vi "runScript.vi"(6 "timeStamp":string, 8 "error in (no error)":errorcluster, 9 "Path":path, 10 "CompiledScript":T1, 11 "AtomChipHWC in":refnum<class "AtomChipHWC.lvclass">) -> (0 "error out":errorcluster, 3 "AtomChipHWC out":refnum<class "AtomChipHWC.lvclass">)   [LabVIEW 2011, in "Hardware.lvlib" / "HWControllers.lvlib" / "AtomChipHWC.lvclass"]
uses:
  AtomChipHWC.lvclass
  Tools/SettingsProcessors/ScriptListCompiler/ScriptListCompiler.lvclass
  Channels/VoltOutput/AnalogOutput.lvclass
  Channels/Digital/DigitalOutput.lvclass
  Channels/DDSOutput/Generic/DDSOutput.lvclass
  AtomChipHWC.lvclass/AtomChipHWC.ctl
  HWController.lvclass
  HardwareConfiguration/HWConfiguration.lvclass
panel:
  out "Analog time":dbl
  out "DDS time":dbl
  out "Digital Time":dbl
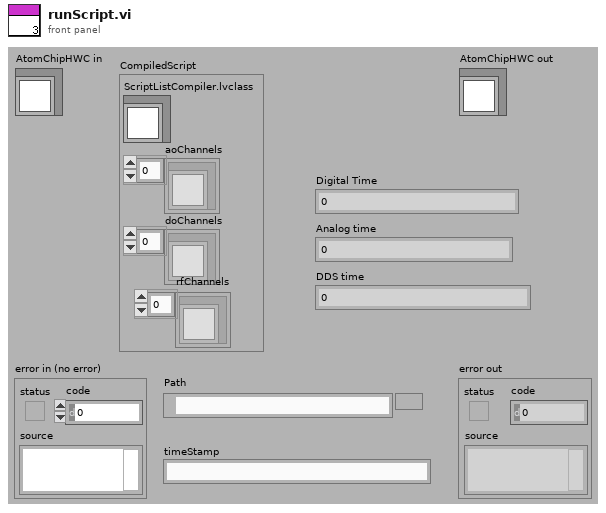
[diagram p1: front panel]
types:
  T1 = cluster{"ScriptListCompiler.lvclass":refnum<class "ScriptListCompiler.lvclass">, "aoChannels":refnum<class "AnalogOutput.lvclass">[], "doChannels":refnum<class "DigitalOutput.lvclass">[], "rfChannels":refnum<class "DDSOutput.lvclass">[]}
  T2 = enum16{"Ready", "Compiling", "Configured", "Running", "Stopping", "Unresolved Error"}
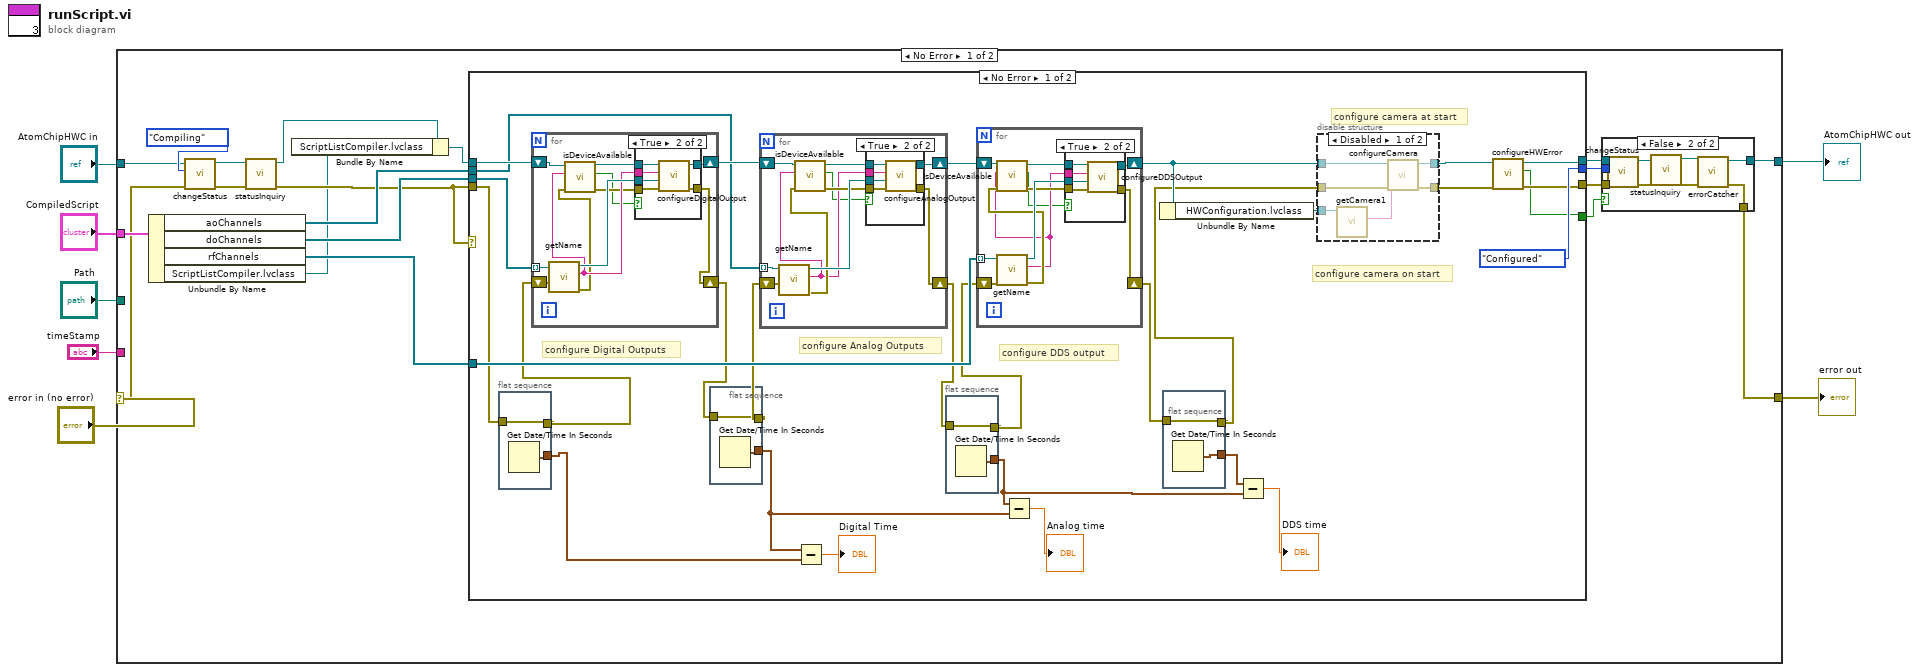
[diagram p0: block diagram]
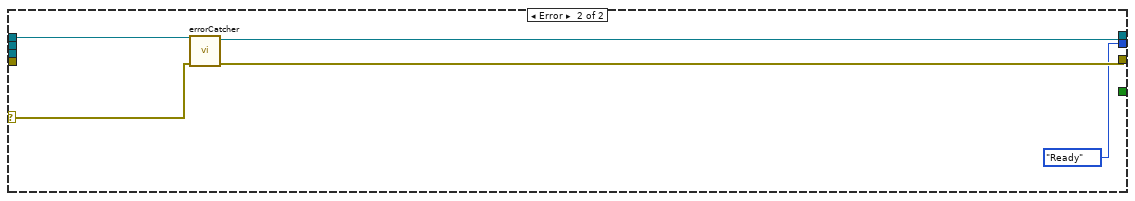
[diagram p7: hidden frame]
diagram:
  n1 = case shown="No Error" "error in (no error)" {
    selector: "error in (no error)" -> [w12 w145]
    tunnel: "AtomChipHWC in" -> [w13 w146]
    tunnel: [w17 w146] -> w5
    tunnel: [w16 w145] -> w4
    tunnel: "CompiledScript" -> [w20 _]
    tunnel: "timeStamp" -> [_ _]
    tunnel: "Path" -> [_ _]
    frame No Error {
      n2 = Unbundle By Name(w20) -> ("aoChannels"=w18:refnum<class "AnalogOutput.lvclass">[], "doChannels"=w19:refnum<class "DigitalOutput.lvclass">[], "rfChannels"=w15:refnum<class "DDSOutput.lvclass">[], "ScriptListCompiler.lvclass"=w8:refnum<class "ScriptListCompiler.lvclass">)
      n3 = call "changeStatus.vi"("error in (no error)"=w12, "status"=T2."Compiling", "HWController in"=w13) -> ("error out"=w24:errorcluster, "HWController out"=w23:refnum<class "AtomChipHWC.lvclass">)  [unwired: 7 in]
      n4 = call-dynamic "statusInquiry.vi"("error in (no error)"=w24, "HWController in"=w23) -> ("error out"=w11:errorcluster, "HWController out"=w10:refnum<class "AtomChipHWC.lvclass">)  [unwired: 8 in]
      n5 = Bundle By Name(cluster=w10, "ScriptListCompiler.lvclass"=w8) -> (w9:refnum<class "AtomChipHWC.lvclass">)
      n6 = case shown="No Error" w11 {
        selector: w11 -> [_ w141]
        tunnel: [w54 w143] -> w26
        tunnel: [w55 w142] -> w25
        tunnel: w9 -> [w65 w144]
        tunnel: w11 -> [w52 _]
        tunnel: w19 -> [w64 _]
        tunnel: w18 -> [w63 _]
        tunnel: [T2."Configured" ("status") T2."Ready" ("status")] -> w21
        tunnel: w15 -> [w61 _]
        tunnel: [w53 _] -> w14
        frame No Error {
          # "configure DDS output"
          # "configure camera at start"
          # "configure camera on start"
          # "configure Analog Outputs"
          # "configure Digital Outputs"
          n7 = flat-sequence {
            tunnel: [w74] -> w51
            tunnel: w52 -> [w74]
            tunnel: [w73] -> w46
            frame #0 {
              n8 = Get Date/Time In Seconds() -> (seconds since 1Jan1904=w73:timestamp)
            }
          }
          n9 = for {
            shift-right: [w128] -> w50
            shift-left: w51 -> [w131]
            shift-right: [w130] -> w66
            shift-left: w65 -> [w126]
            tunnel: w64 -> [w127] mode=indexing
            n10 = call-dynamic "getName.vi"("error in (no error)"=w131, "DigitalOutput.lvclass in"=w127) -> ("error out"=w124:errorcluster, "name"=w125:string, "DigitalOutput.lvclass out"=w129:refnum<class "DigitalOutput.lvclass">)  [unwired: 7 in]
            n11 = call "isDeviceAvailable.vi"("error in (no error)"=w124, "device"=w125, "HWController in"=w126) -> ("error out"=w123:errorcluster, "available"=w121:bool, "HWController out"=w122:refnum<class "AtomChipHWC.lvclass">)  [unwired: 6 in]
            n12 = case shown="True" w121 {
              tunnel: [w133 w139] -> w130
              tunnel: w129 -> [_ w138]
              tunnel: [w132 w137] -> w128
              tunnel: w125 -> [_ w136]
              tunnel: w123 -> [w132 w135]
              tunnel: w122 -> [w133 w134]
              frame False {
              }
              frame True {
                n13 = call "configureDigitalOutput.vi"("error in (no error)"=w135, "DigitalOutput"=w138, "deviceName"=w136, "AtomChipHWC in"=w134) -> ("error out"=w137:errorcluster, "AtomChipHWC out"=w139:refnum<class "AtomChipHWC.lvclass">)  [unwired: 6 in]
              }
            }
          }
          n14 = flat-sequence {
            tunnel: [w72] -> w49
            tunnel: w50 -> [w72]
            tunnel: [w71] -> w44
            frame #0 {
              n15 = Get Date/Time In Seconds() -> (seconds since 1Jan1904=w71:timestamp)
            }
          }
          n16 = for {
            tunnel: w63 -> [w108] mode=indexing
            shift-right: [w110] -> w48
            shift-left: w49 -> [w112]
            shift-right: [w111] -> w60
            shift-left: w66 -> [w107]
            n17 = call "getName.vi"("error in (no error)"=w112, "AnalogOutput.lvclass in"=w108) -> ("error out"=w106:errorcluster, "name"=w103:string, "AnalogOutput.lvclass out"=w109:refnum<class "AnalogOutput.lvclass">)  [unwired: 7 in]
            n18 = call "isDeviceAvailable.vi"("error in (no error)"=w106, "device"=w103, "HWController in"=w107) -> ("error out"=w105:errorcluster, "available"=w102:bool, "HWController out"=w104:refnum<class "AtomChipHWC.lvclass">)  [unwired: 6 in]
            n19 = case shown="True" w102 {
              tunnel: [w114 w120] -> w111
              tunnel: [w113 w119] -> w110
              tunnel: w109 -> [_ w118]
              tunnel: w105 -> [w113 w117]
              tunnel: w104 -> [w114 w116]
              tunnel: w103 -> [_ w115]
              frame False {
              }
              frame True {
                n20 = call "configureAnalogOutput.vi"("error in (no error)"=w117, "AnalogOutput"=w118, "deviceName"=w115, "AtomChipHWC in"=w116) -> ("error out"=w119:errorcluster, "AtomChipHWC out"=w120:refnum<class "AtomChipHWC.lvclass">)  [unwired: 6 in]
              }
            }
          }
          n21 = Subtract(x=w44, y=w46) -> (x-y=→"Digital Time":dbl)
          n22 = flat-sequence {
            tunnel: [w70] -> w47
            tunnel: w48 -> [w70]
            tunnel: [w69] -> w40
            frame #0 {
              n23 = Get Date/Time In Seconds() -> (seconds since 1Jan1904=w69:timestamp)
            }
          }
          n24 = for {
            tunnel: w61 -> [w93] mode=indexing
            shift-right: [w90] -> w43
            shift-left: w47 -> [w92]
            shift-right: [w91] -> w59
            shift-left: w60 -> [w85]
            n25 = call-dynamic "getName.vi"("error in (no error)"=w92, "DDSOutput in"=w93) -> ("error out"=w87:errorcluster, "name"=w86:string, "DDSOutput out"=w89:refnum<class "DDSOutput.lvclass">)  [unwired: 7 in]
            n26 = call "isDeviceAvailable.vi"("error in (no error)"=w87, "device"=w86, "HWController in"=w85) -> ("error out"=w88:errorcluster, "available"=w83:bool, "HWController out"=w84:refnum<class "AtomChipHWC.lvclass">)  [unwired: 6 in]
            n27 = case shown="True" w83 {
              tunnel: [w95 w101] -> w91
              tunnel: [w94 w100] -> w90
              tunnel: w89 -> [_ w99]
              tunnel: w88 -> [w94 w98]
              tunnel: w86 -> [_ w97]
              tunnel: w84 -> [w95 w96]
              frame False {
              }
              frame True {
                n28 = call "configureDDSOutput.vi"("error in (no error)"=w98, "DDSOutput"=w99, "device"=w97, "AtomChipHWC in"=w96) -> ("error out"=w100:errorcluster, "AtomChipHWC out"=w101:refnum<class "AtomChipHWC.lvclass">)  [unwired: 6 in]
              }
            }
          }
          n29 = Subtract(x=w40, y=w44) -> (x-y=→"Analog time":dbl)
          n30 = Unbundle By Name(w59) -> ("HWConfiguration.lvclass"=w58:refnum<class "HWConfiguration.lvclass">)
          n31 = flat-sequence {
            tunnel: [w68] -> w42
            tunnel: w43 -> [w68]
            tunnel: [w67] -> w41
            frame #0 {
              n32 = Get Date/Time In Seconds() -> (seconds since 1Jan1904=w67:timestamp)
            }
          }
          n33 = Subtract(x=w41, y=w40) -> (x-y=→"DDS time":dbl)
          n34 = disable-structure shown="Disabled" {
            disable-tunnel: w42 -> [w80 w81]
            disable-tunnel: [w79 w82] -> w57
            disable-tunnel: [w78 w81] -> w56
            disable-tunnel: w59 -> [w77 w82]
            disable-tunnel: w58 -> [w76 _]
            frame Disabled {
              n35 = call-dynamic "getCamera1.vi"("HWConfiguration.lvclass in"=w76) -> ("camera1"=w75:string)  [unwired: 8 in, 2 out]
              n36 = call "configureCamera.vi"("error in (no error)"=w80, "device"=w75, "AtomChipHWC in"=w77) -> ("error out"=w78:errorcluster, "AtomChipHWC out"=w79:refnum<class "AtomChipHWC.lvclass">)  [unwired: 7 in]
            }
            frame Enabled {
            }
          }
          n37 = call-dynamic "configureHWError.vi"("error in (no error)"=w56, "AtomChipHWC in"=w57) -> ("error out"=w55:errorcluster, "error"=w53:bool, "AtomChipHWC out"=w54:refnum<class "AtomChipHWC.lvclass">)  [unwired: 7 in]
        }
        frame Error {
          n38 = call-dynamic "errorCatcher.vi"("error in (no error)"=w141, "HWController in"=w144) -> ("error out"=w142:errorcluster, "HWController out"=w143:refnum<class "AtomChipHWC.lvclass">)  [unwired: 8 in]
        }
      }
      n39 = case shown="False" w14 {
        tunnel: w26 -> [w28 w37]
        tunnel: w25 -> [w27 w36]
        tunnel: w21 -> [_ w33]
        tunnel: [w28 w30] -> w17
        tunnel: [w27 w29] -> w16
        frame True {
        }
        frame False {
          n40 = call "changeStatus.vi"("error in (no error)"=w36, "status"=w33, "HWController in"=w37) -> ("error out"=w35:errorcluster, "HWController out"=w34:refnum<class "AtomChipHWC.lvclass">)  [unwired: 7 in]
          n41 = call-dynamic "statusInquiry.vi"("error in (no error)"=w35, "HWController in"=w34) -> ("error out"=w31:errorcluster, "HWController out"=w32:refnum<class "AtomChipHWC.lvclass">)  [unwired: 8 in]
          n42 = call-dynamic "errorCatcher.vi"("error in (no error)"=w31, "HWController in"=w32) -> ("error out"=w29:errorcluster, "HWController out"=w30:refnum<class "AtomChipHWC.lvclass">)  [unwired: 8 in]
        }
      }
    }
    frame Error {
    }
  }
  "error out" <- w4
  "AtomChipHWC out" <- w5
